vi "Memory.Pointer.Clear.Safe.vi"(8 "error in (no error)":errorcluster, 11 "pointer in":refnum<class "Memory.Pointer.lvclass">) -> (0 "error out":errorcluster, 3 "pointer out":refnum<class "Memory.Pointer.lvclass">)   [LabVIEW 2016, in "Memory.lvlib" / "Memory.Pointer.lvclass"]
doc: "Sets all of the bytes specified by <b>pointer</b> to zero.\n\n<b>Note:</b> This VI is <b>safe</b>, meaning it performs null pointer and bounds checks to prevent invaid memory access."
uses:
  Memory.Pointer.lvclass
  Memory.Pointer.lvclass/Memory.Pointer.ctl
  Memory.Pointer.Errors.vi
  Memory.Pointer.Errors.Null Pointer.vi
  Memory.Pointer.Get Address.vi
  Memory.Pointer.Clear Subset.Unsafe.vi
  Memory.Pointer.Errors.Create Error.vi
  Memory.Pointer.Get Size.vi
  Submodules/SEH/Source/VIs/Static Error Handling.Error Cluster Constant.vi
  Submodules/SEH/Source/VIs/Static Error Handling.Error Cluster Constant (256B).vi
  Submodules/SEH/Source/VIs/Static Error Handling.Parameters.Status.Set.vi
  Submodules/SEH/Source/VIs/Static Error Handling.Parameters.Code.Set.vi
  Submodules/SEH/Source/VIs/Static Error Handling.Parameters.VI Source.Set.vi
  Constants/Memory.Constants.vi
  Constants/Memory.Constants.Library Name.vi
  Memory.Pointer.Errors.Get Info.vi
  Submodules/SEH/Source/VIs/Static Error Handling.Source Buffer.Write.String.vi
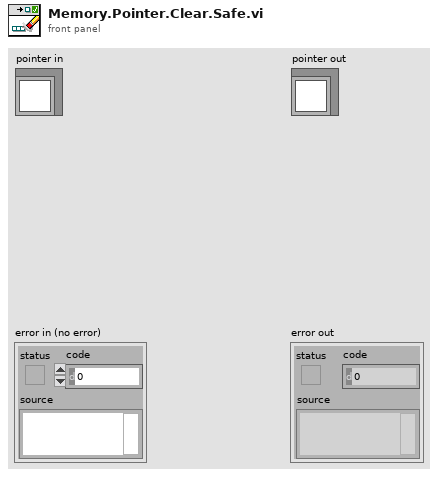
[diagram p1: front panel]
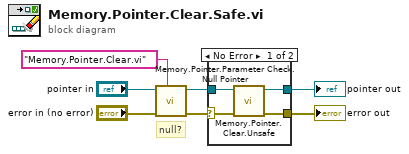
[diagram p0: block diagram]
diagram:
  # "null?"
  n1 = call "Memory.Pointer.Parameter Check.Null Pointer.vi"("source vi name"="Memory.Pointer.Clear.vi", "error in (no error)"="error in (no error)", "Pointer in"="pointer in") -> ("error out"=w1:errorcluster, "Pointer out"=w4:refnum<class "Memory.Pointer.lvclass">)  [unwired: 7 in]
  n2 = case shown="No Error" w1 {
    selector: w1 -> [w8 w13]
    tunnel: w4 -> [w11 w12]
    tunnel: [w10 w12] -> w3
    tunnel: [w9 w13] -> w2
    frame No Error {
      n3 = call "Memory.Pointer.Clear.Unsafe.vi"("error in (no error)"=w8, "pointer in"=w11) -> ("error out"=w9:errorcluster, "pointer out"=w10:refnum<class "Memory.Pointer.lvclass">)  [unwired: 8 in]
    }
    frame Error {
    }
  }
  "error out" <- w2
  "pointer out" <- w3
